vi "Antenna Test.vi"(9 "Simulation Data":T2={"PowerOn"=TRUE, "Battery"=TRUE, "Antenna"=TRUE, "Microphone"=TRUE, "Speakers"=TRUE, "Buttons"=TRUE, "LCD"=enum."Passing Image"}, 10 "Mode":T1, 11 "Transmitted Data String":string="1. Generate System Parameters.  This VI generates a symbol map and computes bits per symbol for the given QAM selection.\n2. Bit Coding.  This VI converts an array of U8 characters into a binary array, adding Log2(M) guard bits to the front of the bistream.\n3. Generate Filter Coefficients.  Generates pulse shaping and matching filter coefficients\n4. Modulate QAM.  Converts the bitstream into an array of IQ values.\n5. Add AWGN.  This VI adds impairments such as increasing the noise floor of the signal\n    (note, steps 6 and 7 are used only for visualization/analysis purposes)\n6. Upconversion.  Converts an array of IQ values into a waveform based on the carrier frequency\n7. Spectral Measurements.  Performs an FFT of the upconverted waveform to illustrate the carrier band.\n8. Demodulate QAM.  Conerts an array of IQ values into a bitstream\n    (note, step 9 is used only for visualization/analysis purposes)\n9. Format Constillation Plot.  Generate a constilation plot for the demodulated IQ data.\n10. Convert the bistream into an array of U8's, so that that the resulting information can be viewed in character format.\n\nqwertyuiop[asdfghjkl;xcvbnm,./\n") -> (0 "Error Out":errorcluster, 2 "Image Report String":string, 3 "UUT String Received":string)   [LabVIEW 2011]
doc: "Translates the test string into a bitstream, and then encodes it into a QAM signal, which is transmitted using the Tester RFSG. The received signal on the device is then read by the UUT controller and translated back into a string."
uses:
  Support/Simulation Data.ctl
  Support/Wifi Test Modes.ctl
panel:
  out "QAM Data Transmitted":cluster{dbl[], dbl[]}[](graph)
  out "QAM Data Received":cluster{dbl[], dbl[]}[](graph)
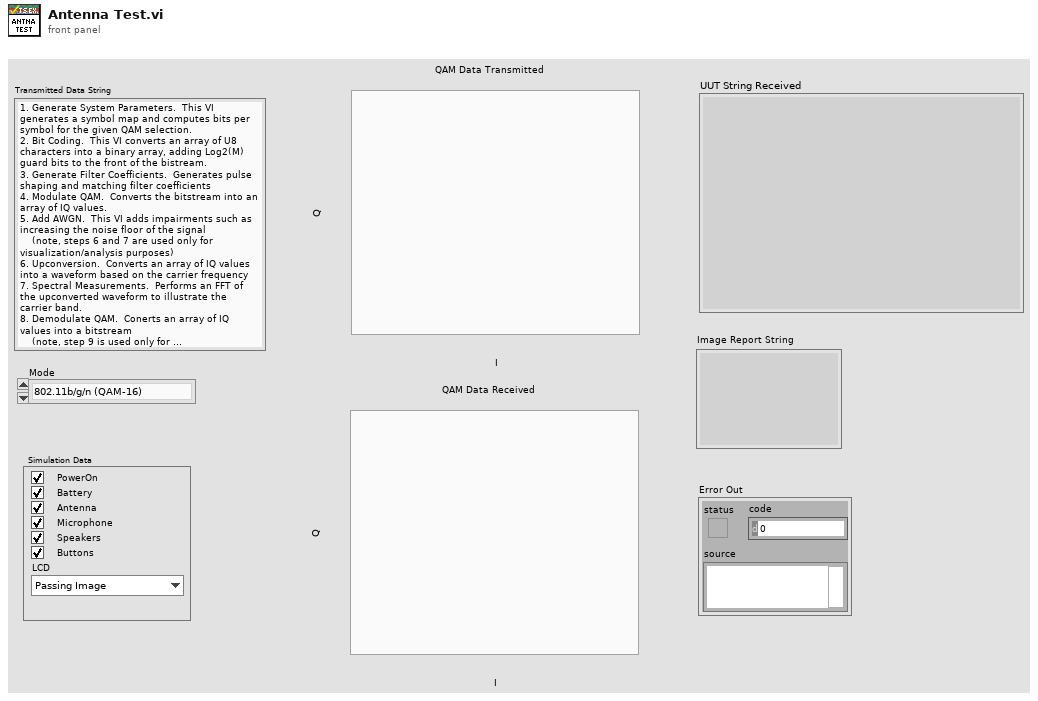
[diagram p1: front panel]
types:
  T1 = typedef "Wifi Test Modes.ctl" = enum16{"802.11b/g/n (QAM-16)", "LTE (QAM-64)", "802.11ac (QAM-256)"}
  T2 = typedef "Simulation Data.ctl" = cluster{"PowerOn":bool, "Battery":bool, "Antenna":bool, "Microphone":bool, "Speakers":bool, "Buttons":bool, "LCD":enum16{"Passing Image", "Dead Pixels", "Incorrect Brightness"}}
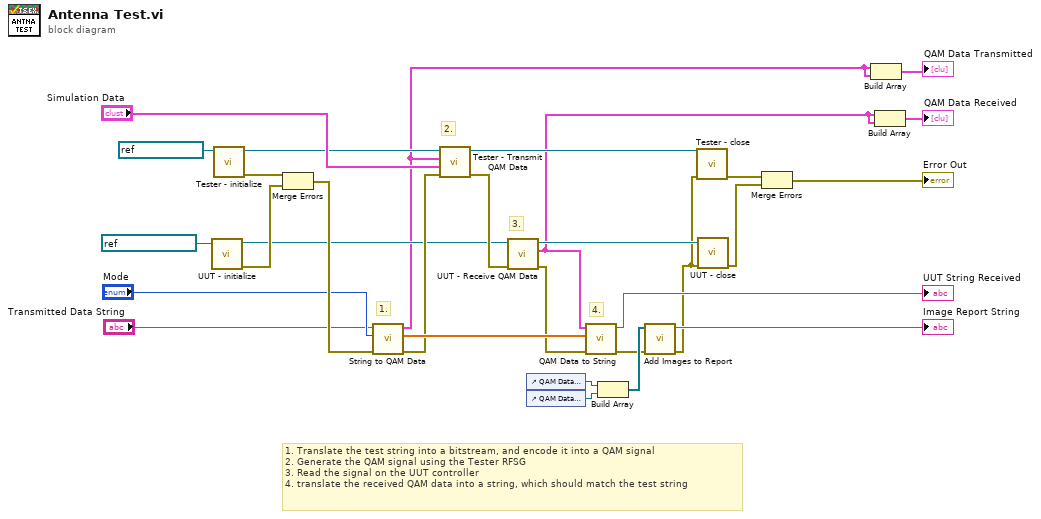
[diagram p0: block diagram]
diagram:
  # "4."
  # "3."
  # "2."
  # "1."
  # "1. Translate the test string into a bitstream, and encode it into a QAM signal\n2. Generate the QAM signal using the Tester RFSG\n3. Read the signal on the UUT controller\n4. translate the received QAM data into a string, which should match the test string"
  n1 = call "UUT - initialize.vi"("VISA resource name"=refnum<visa-resource-name> "UUTController") -> ("error out"=w25:errorcluster, "VISA resource name out"=w18:refnum<visa-resource-name>)  [unwired: 9 in]
  n2 = call "Tester - initialize.vi"("VISA resource name"=refnum<visa-resource-name> "TesterRFSG") -> ("error out"=w27:errorcluster, "VISA resource name out"=w21:refnum<visa-resource-name>)  [unwired: 9 in]
  n3 = Merge Errors(w27, w25) -> (w24:errorcluster)
  n4 = call "String to QAM Data.vi"("error in (no error)"=w24, "Mode"="Mode", "Transmitted Data String"="Transmitted Data String") -> ("error out"=w22:errorcluster, "symbol map 16 QAM"=w30:cdb[], "QAM Data"=w3:cluster{dbl[], dbl[]})  [unwired: 6 in]
  n5 = call "Tester - Transmit QAM Data.vi"("error in (no error)"=w22, "Simulation Data"="Simulation Data", "QAM Data In"=w3, "VISA resource name"=w21) -> ("error out"=w19:errorcluster, "VISA resource name out"=w14:refnum<visa-resource-name>)  [unwired: 6 in]
  n6 = call "UUT - Receive QAM Data.vi"("error in (no error)"=w19, "VISA resource name"=w18) -> ("error out"=w20:errorcluster, "QAM Data Out"=w2:cluster{dbl[], dbl[]}, "VISA resource name out"=w15:refnum<visa-resource-name>)  [unwired: 7 in]
  n7 = control-ref of="QAM Data Received"() -> (w13:refnum<vi>)
  n8 = control-ref of="QAM Data Transmitted"() -> (w12:refnum<vi>)
  n9 = call "QAM Data to String.vi"("error in (no error)"=w20, "symbol map 16 QAM"=w30, "QAM Data Out"=w2) -> ("error out"=w9:errorcluster, "Output String"=→"UUT String Received":string)  [unwired: 7 in]
  n10 = Build Array(w13, w12) -> (w11:refnum<vi>[])
  n11 = call "Add Images to Report.vi"("error in (no error)"=w9, "Control References"=w11) -> ("error out"=w8:errorcluster, "Report String"=→"Image Report String":string)  [unwired: 8 in]
  n12 = call "Tester - close.vi"("error in (no error)"=w8, "VISA resource name"=w14) -> ("error out"=w16:errorcluster)  [unwired: 9 in]
  n13 = call "UUT - close.vi"("error in (no error)"=w8, "VISA resource name"=w15) -> ("error out"=w17:errorcluster)  [unwired: 9 in]
  n14 = Merge Errors(w16, w17) -> (→"Error Out":errorcluster)
  n15 = Build Array(w3, w3) -> (→"QAM Data Transmitted":cluster{dbl[], dbl[]}[])
  n16 = Build Array(w2, w2) -> (→"QAM Data Received":cluster{dbl[], dbl[]}[])
